vi "Configure Frequency (Reflection Measurement - Start Stop).vi"(0 "VISA resource name":refnum<visa-resource-name>, 5 "Start Frequency (5E+6 Hz)":dbl=5000000.0, 9 "Stop Frequency (5E+8 Hz)":dbl=500000000.0, 11 "error in (no error)":errorcluster) -> (4 "VISA resource name out":refnum<visa-resource-name>, 15 "error out":errorcluster)   [LabVIEW 2022 SP3, in "Agilent N934X Series.lvlib"]
doc: "Configure the start stop frequency of Reflection Measurement type.\n\nNote:\nThis VI is only applicable for N9321C, N9322C, N9323C, N9324C models."
uses:
  <instrlib>/Agilent N934X Series/Agilent N934X Series.lvlib
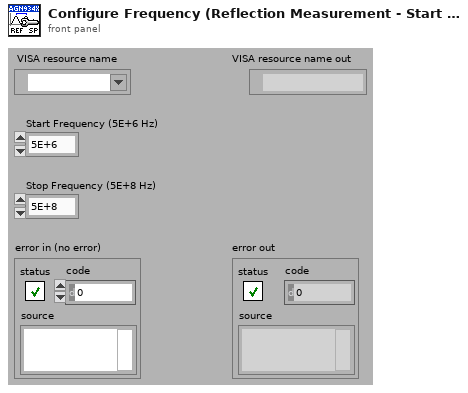
[diagram p1: front panel]
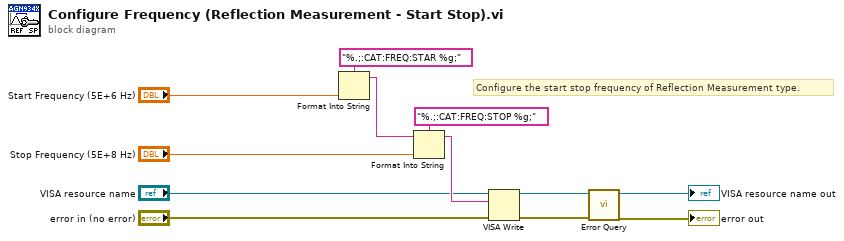
[diagram p0: block diagram]
diagram:
  # "Configure the start stop frequency of Reflection Measurement type."
  n1 = Format Into String(format string="%.;:CAT:FREQ:STAR %g;", "Start Frequency (5E+6 Hz)") -> (resulting string=w10:string)  [unwired: 2 in, 1 out]
  n2 = Format Into String(format string="%.;:CAT:FREQ:STOP %g;", initial string=w10, "Stop Frequency (5E+8 Hz)") -> (resulting string=w7:string)  [unwired: 1 in, 1 out]
  n3 = VISA Write(VISA resource name="VISA resource name", write buffer=w7, error in (no error)="error in (no error)") -> (VISA resource name out=w4:refnum<visa-resource-name>, error out=w3:errorcluster)  [unwired: 1 out]
  n4 = call <instrlib>:"Error Query.vi"("error in (no error)"=w3, "VISA resource name"=w4) -> ("error out"=→"error out":errorcluster, "VISA resource name out"=→"VISA resource name out":refnum<visa-resource-name>)  [unwired: 6 in, 2 out]
